vi "1HzN2Hz.vi"() -> ()   [LabVIEW 2015]
panel:
  in  "stop":bool
  out "LED1 (1Hz)":bool
  out "LED2 (2Hz)":bool
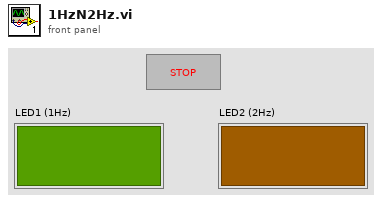
[diagram p1: front panel]
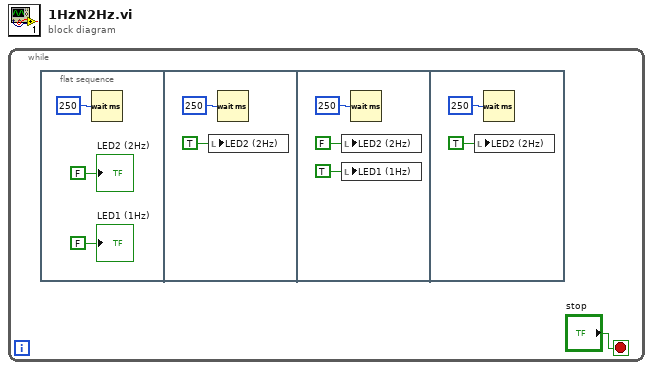
[diagram p0: block diagram]
diagram:
  n1 = while {
    stop <- "stop" stop-if-true
    n2 = flat-sequence {
      frame #0 {
        n3 = Wait (ms)(milliseconds to wait=u32 250) -> ()  [unwired: 1 out]
        "LED2 (2Hz)" <- FALSE ("Boolean")
        "LED1 (1Hz)" <- FALSE ("Boolean 2")
      }
      frame #1 {
        n4 = local write "LED2 (2Hz)"(TRUE) -> ()
        n5 = Wait (ms)(milliseconds to wait=u32 250) -> ()  [unwired: 1 out]
      }
      frame #2 {
        n6 = local write "LED2 (2Hz)"(FALSE) -> ()
        n7 = local write "LED1 (1Hz)"(TRUE) -> ()
        n8 = Wait (ms)(milliseconds to wait=u32 250) -> ()  [unwired: 1 out]
      }
      frame #3 {
        n9 = local write "LED2 (2Hz)"(TRUE) -> ()
        n10 = Wait (ms)(milliseconds to wait=u32 250) -> ()  [unwired: 1 out]
      }
    }
  }
